vi "Fit.vi"(7 "Type X":T1(ring), 8 "error in (no error)":errorcluster caption="entrée d'erreur (pas d'erreur)", 9 "y":string[][](array[string]), 10 "X":string[][](array[string]), 11 "RBFSampler.lvclass":refnum<class "RBFSampler.lvclass">) -> (0 "error out":errorcluster caption="sortie d'erreur", 2 "String Data":string, 3 "RBFSampler.lvclass":refnum<class "RBFSampler.lvclass">)   [LabVIEW 2020, in "RBFSampler.lvclass"]
doc: "Fit the model with X.\n\nSamples random projection according to n_features.\n\nReturns : \n\n- String : OK"
uses:
  RBFSampler.lvclass
  RBFSampler.lvclass/RBFSampler.ctl
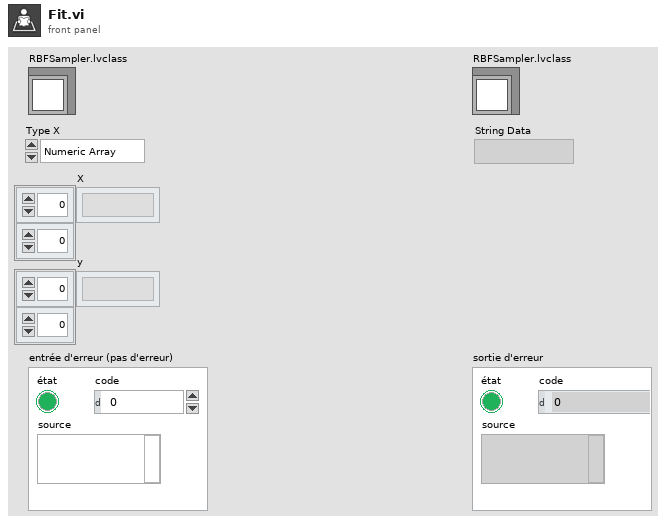
[diagram p1: front panel]
types:
  T1 = enum16{"Numeric Array", "String Array", "Sparse"}
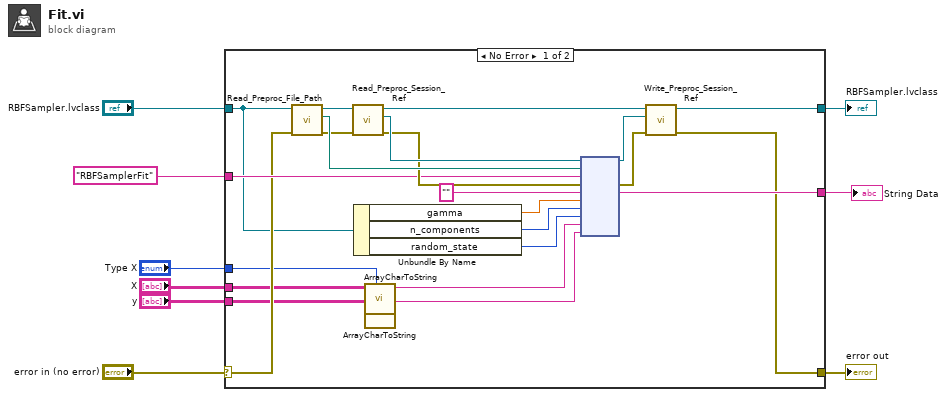
[diagram p0: block diagram]
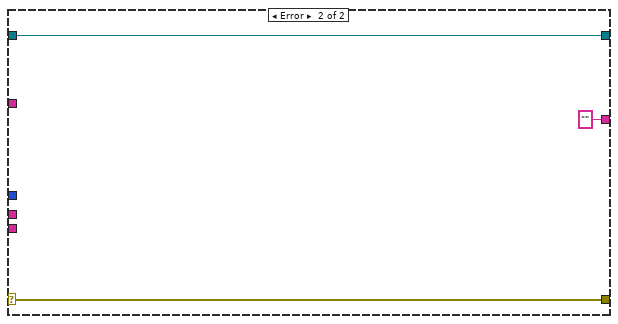
[diagram p2: hidden frame]
diagram:
  n1 = case shown="No Error" "error in (no error)" {
    selector: "error in (no error)" -> [w20 w35]
    tunnel: [w16 w35] -> w8
    tunnel: [w18 w34] -> w6
    tunnel: "RBFSampler.lvclass" -> [w17 w34]
    tunnel: "RBFSamplerFit" ("Fonction") -> [w21 _]
    tunnel: "X" -> [w14 _]
    tunnel: [w19 ""] -> w3
    tunnel: "y" -> [w12 _]
    tunnel: "Type X" -> [w10 _]
    frame No Error {
      n2 = call-dynamic "Read_Preproc_File_Path.vi"("error in (no error)"=w20, "Python in"=w17) -> ("error out"=w27:errorcluster, "File_Path"=w30:path, "Python out"=w32:refnum<class "RBFSampler.lvclass">)  [unwired: 7 in]
      n3 = call-dynamic "Read_Preproc_Session_Ref.vi"("error in (no error)"=w27, "Python in"=w32) -> ("error out"=w28:errorcluster, "Session_ref"=w29:refnum<k35>, "Python out"=w31:refnum<class "RBFSampler.lvclass">)  [unwired: 7 in]
      n4 = Unbundle By Name(w17) -> ("gamma"=w23:dbl, "n_components"=w22:i32, "random_state"=w15:i32)
      n5 = call "ArrayCharToString.vi"("Type"=w10, "TAB"=w14) -> ("Instruction"=w13:string)  [unwired: 9 in]
      n6 = call "ArrayCharToString.vi"("TAB"=w12) -> ("Instruction"=w11:string)  [unwired: 10 in]
      n7 = node(w29, w30, w21, w28, "", w23, w22, w15, w13, w11) -> (w24:refnum<k35>, w26:errorcluster, w19:string)  [unwired: 5 in, 2 out]
      n8 = call-dynamic "Write_Preproc_Session_Ref.vi"("error in (no error)"=w26, "Session_ref"=w24, "Python in"=w31) -> ("error out"=w16:errorcluster, "Python out"=w18:refnum<class "RBFSampler.lvclass">)  [unwired: 7 in]
    }
    frame Error {
    }
  }
  "error out" <- w8
  "RBFSampler.lvclass" <- w6
  "String Data" <- w3
